vi "OAT FIR Preprocess Filter.vi"   [LabVIEW 2017, in "SoundVib_RefDataProcess.lvlib"]
doc: "Designs an FIR filter and filters the <B>scaled signal [EU]</B>. Wire data to the <B>scaled signal [EU]</B> input to determine the polymorphic instance to use or manually select the instance."
uses:
  <vilib>/addons/Sound and Vibration/Order Analysis/Referece Data Processing/SoundVib_RefDataProcess.lvlib
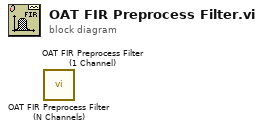
[diagram p0: block diagram]
diagram:
  n1 = call <vilib>:"OAT FIR Preprocess Filter (N Channels).vi"() -> ()  [unwired: 13 in, 3 out]
  n2 = call <vilib>:"OAT FIR Preprocess Filter (1 Channel).vi"() -> ()  [unwired: 13 in, 3 out]
